vi "convertToIFontUnderline.vi"(11 "Underline":T1=18 items=["Single"=1, "Words"=2, "Double"=3, "Thick"=4, "Dotted"=5, "DottedHeavy"=6, "Dash"=7, "DashedHeavy"=8, "DashLong"=9, "DashLongHeavy"=10, "DotDash"=11, "DashDotHeavy"=12, "DotDotDash"=13, "DashDotDotHeavy"=14, "Wave"=15, "WavyHeavy"=16, "WavyDouble"=17, "None"=18]) -> (3 "IFont.Underline":u8(ring) items=["None"=0, "Single"=1, "Double"=2, "SingleAccounting"=33, "DoubleAccounting"=34])   [LabVIEW 2020, in "LabVIEW NPOI.lvlib" / "MS-Excel.lvclass"]
uses:
  MS-Excel.lvclass
  Styles/Underline--ring.ctl
  Styles/Styles.lvlib
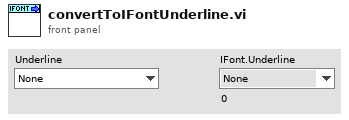
[diagram p1: front panel]
types:
  T1 = typedef "Styles.lvlib/Underline--ring.ctl" = i32
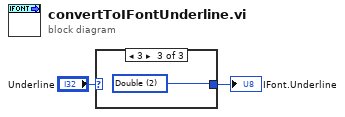
[diagram p0: block diagram]
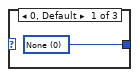
[diagram p2: hidden frame]
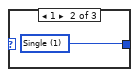
[diagram p3: hidden frame]
diagram:
  n1 = case shown="3" "Underline" {
    tunnel: [w3 w4 w5] -> w1
    frame 0, Default {
      w3 = u8 0 items=["None"=0, "Single"=1, "Double"=2, "SingleAccounting"=33, "DoubleAccounting"=34] ("Underline")
    }
    frame 1 {
      w4 = u8 1 items=["None"=0, "Single"=1, "Double"=2, "SingleAccounting"=33, "DoubleAccounting"=34] ("Underline")
    }
    frame 3 {
      w5 = u8 2 items=["None"=0, "Single"=1, "Double"=2, "SingleAccounting"=33, "DoubleAccounting"=34] ("Underline")
    }
  }
  "IFont.Underline" <- w1
